vi "Wait on Sync Response.vi"(6 "Sync Response":refnum<notifier>, 8 "error in (no error)":errorcluster, 11 "2DArrayManager in":refnum<class "2DArrayManager.lvclass">) -> (0 "error out":errorcluster, 3 "2DArrayManager out":refnum<class "2DArrayManager.lvclass">)   [LabVIEW 2020, in "OOPanel.lvlib" / "2DArrayManager.lvclass"]
uses:
  2DArrayManager.lvclass
panel:
  out "Response Error":errorcluster
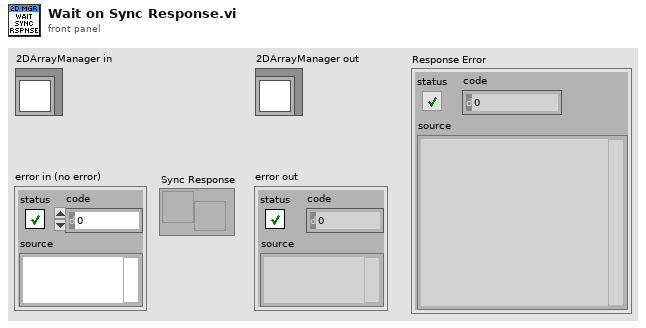
[diagram p1: front panel]
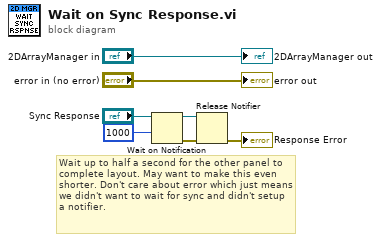
[diagram p0: block diagram]
diagram:
  # "Wait up to half a second for the other panel to complete layout. May want to make this even shorter. Don't care about error which just means we didn't want to wait for sync and didn't setup a notifier."
  n1 = Wait on Notification(notifier="Sync Response", timeout in ms (-1)=1000) -> (notifier out=w3:refnum<notifier>, error out=w2:errorcluster)  [unwired: 2 in, 2 out]
  n2 = Release Notifier(notifier=w3, error in (no error)=w2) -> (error out=→"Response Error":errorcluster)  [unwired: 1 in, 2 out]
  "error out" <- "error in (no error)"
  "2DArrayManager out" <- "2DArrayManager in"
